vi "Destroy.vi"(0 "reference":refnum<class "SequenceDiagramGraph.lvclass">, 5 "error in (no error)":errorcluster) -> (19 "error out":errorcluster)   [LabVIEW 2020, in "SequenceDiagramGraph.lvclass"]
uses:
  <resource>/Framework/Providers/Open_GDS/UML/SequenceDiagramGraph_class/SequenceDiagramGraph.lvclass
  <resource>/Framework/Providers/Open_GDS/UML/Graph_class/Graph.lvclass
panel:
  out "reference out":refnum<class "SequenceDiagramGraph.lvclass">
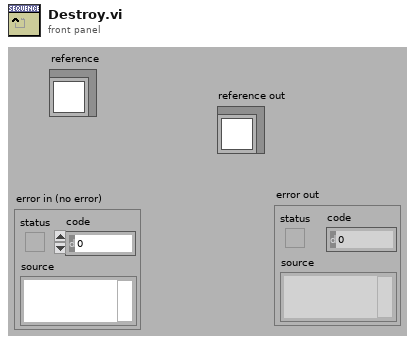
[diagram p1: front panel]
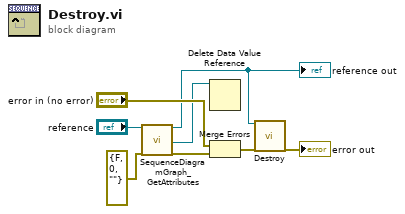
[diagram p0: block diagram]
diagram:
  n1 = call <resource>:"SequenceDiagramGraph_GetAttributes.vi"("reference in"="reference", "error in (no error)"=errorcluster {"status"=FALSE, "code"=0, "source"=""}) -> ("reference out"=w3:refnum<class "SequenceDiagramGraph.lvclass">, "DataRef"=w1:refnum<data-value>, "error out"=w4:errorcluster)  [unwired: 1 in, 14 out]
  "reference out" <- w3
  n2 = Delete Data Value Reference(data value reference=w1) -> ()  [unwired: 1 in, 2 out]
  n3 = Merge Errors("error in (no error)", w4) -> (w2:errorcluster)
  n4 = call-parent "Destroy.vi"("reference"=w3, "error in (no error)"=w2) -> ("error out"=→"error out":errorcluster)  [unwired: 17 in]
